vi "sub build o data.vi"(8 "error in":errorcluster, 11 "<o> data":T1) -> (0 "error out":errorcluster, 3 "<o> string":string)   [LabVIEW 2018, in "Frame Analizer.lvclass"]
uses:
  Frame Analizer.lvclass
  frame o data.ctl
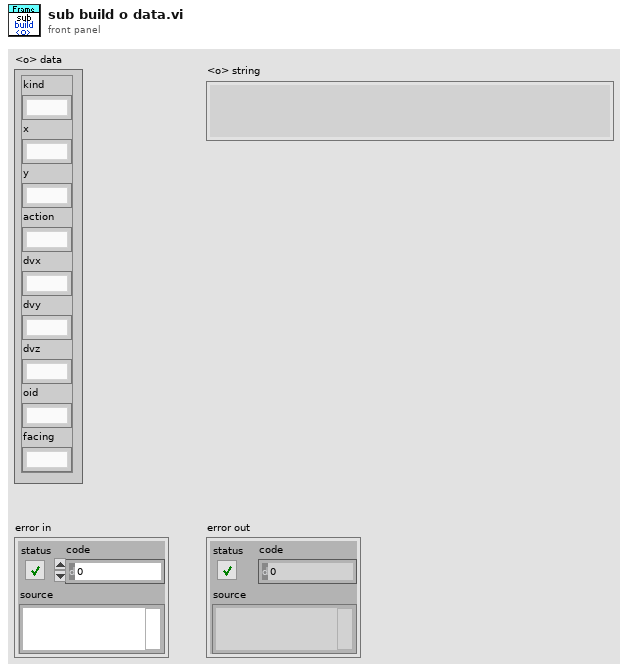
[diagram p1: front panel]
types:
  T1 = typedef "Frame Analizer.lvclass/frame o data.ctl" = cluster{"kind":string, "x":string, "y":string, "action":string, "dvx":string, "dvy":string, "dvz":string, "oid":string, "facing":string}
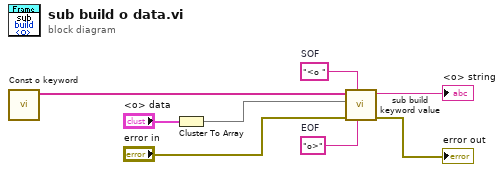
[diagram p0: block diagram]
diagram:
  w4 = "<o "  # SOF
  w2 = "o>"  # EOF
  n1 = call "Const o keyword.vi"() -> ("Const o keyword"=w1:string[])  [unwired: 11 in]
  n2 = Cluster To Array(cluster="<o> data") -> (array=w3:string[])
  n3 = call "sub build keyword value.vi"("EOF"=w2, "SOF"=w4, "error in"="error in", "value"=w3, "keyword"=w1) -> ("error out"=→"error out":errorcluster, "keyword value string"=→"<o> string":string)  [unwired: 5 in]
